vi "write_to_IRM_DB.vi"(2 "error in (no error)":errorcluster, 3 "data":variant, 4 "columns":string[](array[string]), 5 "DB table":string="irm_remanence_measurements") -> (0 "error out":errorcluster)   [LabVIEW 2009]
uses:
  <vilib>/addons/database/Connection.llb/DB Tools Open Connec (String).vi
  DB_Info.vi
  <vilib>/addons/database/NI_Database_API.lvlib
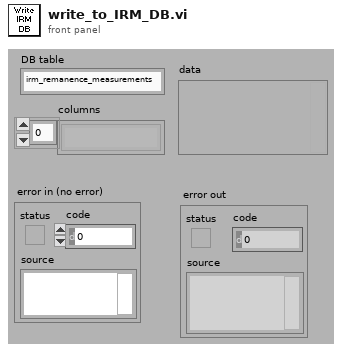
[diagram p1: front panel]
types:
  T1 = typedef "NI_Database_API.lvlib/Conn ObjectReference.ctl" = refnum<k1>
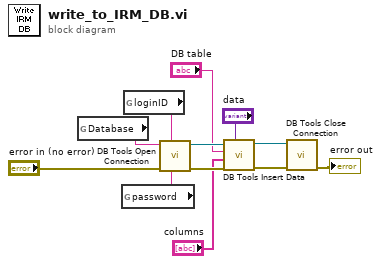
[diagram p0: block diagram]
diagram:
  n1 = global read "DB_Info.vi" "Database"() -> (w2:string)
  n2 = global read "DB_Info.vi" "password"() -> (w3:string)
  n3 = global read "DB_Info.vi" "loginID"() -> (w1:string)
  n4 = call-poly <vilib>:"DB Tools Open Connection.vi"("password"=w3, "userID"=w1, "error in (no error)"="error in (no error)", "connection information"=w2) -> ("error out"=w10:errorcluster, "connection reference"=w9:T1)  [unwired: 1 in, 3 out]
  n5 = call <vilib>:"DB Tools Insert Data.vi"("data"="data", "error in (no error)"=w10, "columns"="columns", "table"="DB table", "connection reference"=w9) -> ("error out"=w7:errorcluster, "connection reference out"=w8:T1)  [unwired: 2 in, 3 out]
  n6 = call <vilib>:"DB Tools Close Connection.vi"("error in (no error)"=w7, "connection reference"=w8) -> ("error out"=→"error out":errorcluster)  [unwired: 5 out]
